vi "PicohrdlUnitInfoSingle.vi"(8 "error in (no error)":errorcluster, 9 "info Enum":i16(ring), 11 "Handle in":i16) -> (0 "error out":errorcluster, 1 "trimmed string":string, 3 "handle out":i16, 6 "status":i16)   [LabVIEW 2010]
doc: "Calls HRDLGetUnitInfo()"
uses:
  PicoHRDL.dll
panel:
  out "stringLength":i16
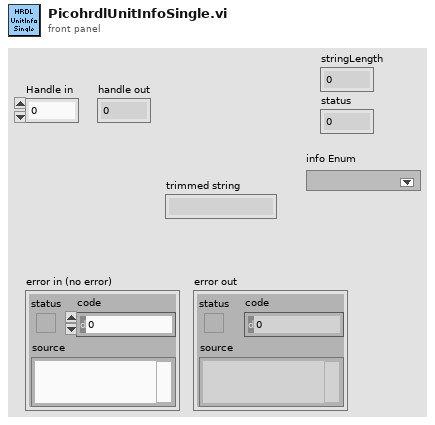
[diagram p1: front panel]
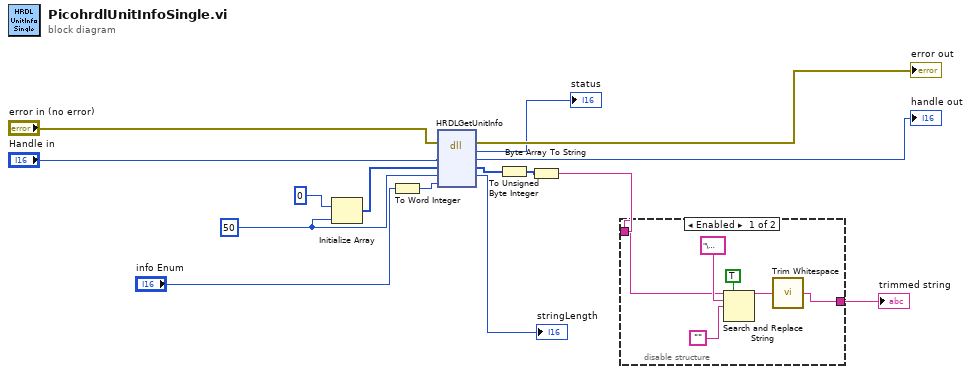
[diagram p0: block diagram]
diagram:
  w7 = i16 50 ("requiredSize")
  n1 = Initialize Array(i8 0 ("element"), w7) -> (w6:i8[])
  n2 = To Word Integer(number="info Enum") -> (16bit integer=w8:i16)
  n3 = dll-call lib="picohrdl.dll" fn="HRDLGetUnitInfo"(error in="error in (no error)", "handle"="Handle in", "unitInfo"=w6, "stringLength"=w7, "info"=w8) -> (error out=→"error out":errorcluster, "status"=→"status":i16, "handle"=→"handle out":i16, "unitInfo"=w5:i8[], "stringLength"=→"stringLength":i16)  [unwired: 3 in, 1 out]
  n4 = To Unsigned Byte Integer(number=w5) -> (unsigned 8bit integer=w15:u8[])
  n5 = Byte Array To String(unsigned byte array=w15) -> (string=w13:string)
  n6 = disable-structure shown="Enabled" {
    disable-tunnel: w13 -> [w17 w22]
    disable-tunnel: [w16 w22] -> w12
    frame Enabled {
      n7 = Search and Replace String(replace all?=TRUE ("replace all? (F)"), input string=w17, search string="\u0000", replace string="") -> (result string=w19:string)  [unwired: 4 in, 3 out]
      n8 = call <vilib>:"Trim Whitespace.vi"("string"=w19) -> ("trimmed string"=w16:string)  [unwired: 1 in]
    }
    frame Disabled {
    }
  }
  "trimmed string" <- w12
